vi "坐标旋转2.vi"(10 "旋转角度(单位弧度)":dbl, 11 "dtx,dty In":cluster{"X":dbl, "Y":dbl}) -> (3 "dtx,dty Out":cluster{"X":dbl, "Y":dbl})   [LabVIEW 2014]
panel:
  out "旋转角度(单位弧度) 2":dbl
  out "x/y":dbl
  out "cos(x)":dbl
  out "sin(x)":dbl
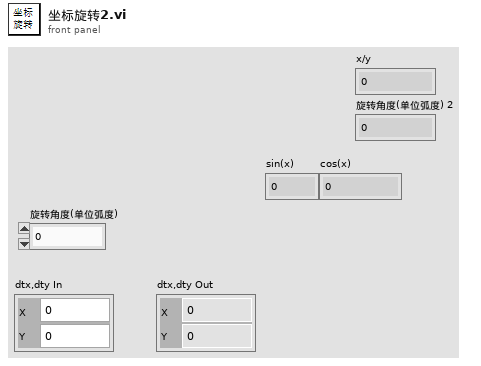
[diagram p1: front panel]
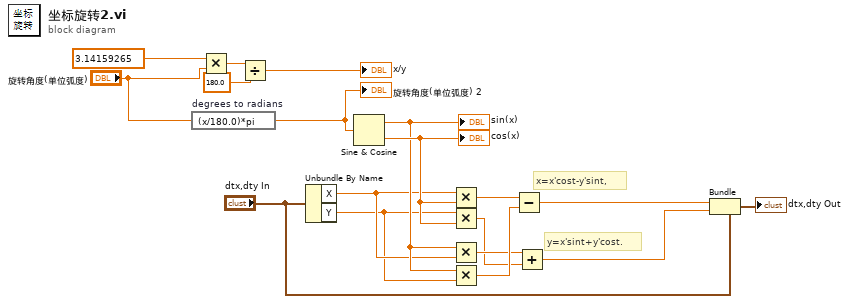
[diagram p0: block diagram]
diagram:
  # "y=x'sint+y'cost."
  # "x=x'cost-y'sint,"
  n1 = expression code="(x/180.0)*pi" "degrees to radians"("旋转角度(单位弧度)") -> (w3:dbl)
  "旋转角度(单位弧度) 2" <- w3
  n2 = Multiply(x=3.14159265, y="旋转角度(单位弧度)") -> (x*y=w5:dbl)
  n3 = Divide(x=w5, y=180.0) -> (x/y=→"x/y":dbl)
  n4 = Unbundle By Name("dtx,dty In") -> ("X"=w16:dbl, "Y"=w15:dbl)
  n5 = Sine & Cosine(0:w3) -> (1:w17:dbl, 2:w18:dbl)
  "sin(x)" <- w17
  "cos(x)" <- w18
  n6 = Multiply(x=w16, y=w18) -> (x*y=w14:dbl)
  n7 = Multiply(x=w15, y=w18) -> (x*y=w11:dbl)
  n8 = Multiply(x=w17, y=w16) -> (x*y=w12:dbl)
  n9 = Multiply(x=w17, y=w15) -> (x*y=w13:dbl)
  n10 = Subtract(x=w14, y=w13) -> (x-y=w10:dbl)
  n11 = Add(x=w12, y=w11) -> (x+y=w9:dbl)
  n12 = Bundle(cluster="dtx,dty In", "X"=w10, "Y"=w9) -> (→"dtx,dty Out":cluster{"X":dbl, "Y":dbl})
